vi "Test Modes.vi"(8 "error in (no error)":errorcluster, 11 "Instrument.Lockin in":refnum<class "Instrument.Lockin.lvclass">) -> (0 "error out":errorcluster, 3 "Instrument.Lockin out":refnum<class "Instrument.Lockin.lvclass">)   [LabVIEW 2016]
uses:
  src/Instrument.Lockin/Instrument.Lockin.lvclass
  src/Lockin.DAQ/Typedefs/AO_Channel-Numeric.ctl
  <vilib>/addons/_JKI Toolkits/Caraya/classes/Assert/Assert Equal Value_Variant.vi
  <vilib>/addons/_JKI Toolkits/Caraya/classes/Assert/Assert Not Error.vi
  <vilib>/addons/_JKI Toolkits/Caraya/classes/Assert/Assert Not Equal Value and Type_Variant.vi
  <vilib>/addons/_JKI Toolkits/Caraya/classes/Test/Test.lvclass
  <vilib>/addons/_JKI Toolkits/Caraya/classes/Assert/Assert.lvclass
  src/Lockin.DAQ/Lockin.DAQ.lvclass
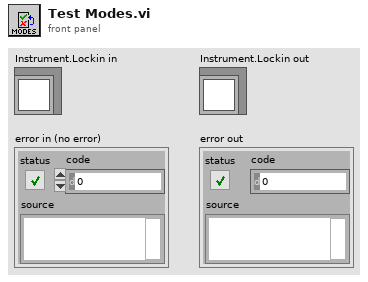
[diagram p1: front panel]
types:
  T1 = typedef "Lockin.DAQ.lvclass/AO_Channel-Numeric.ctl" = i32
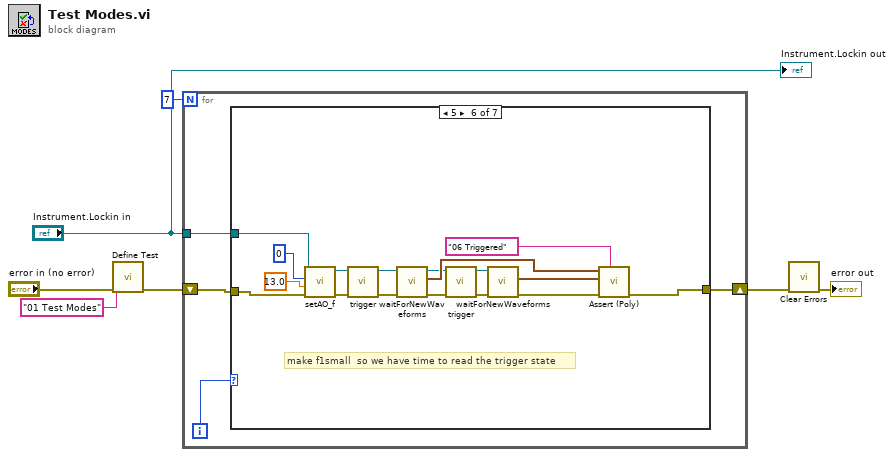
[diagram p0: block diagram]
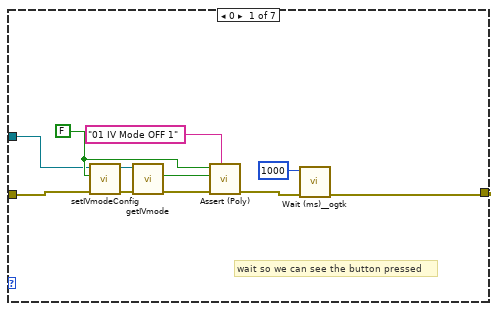
[diagram p2: hidden frame]
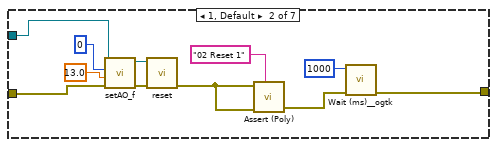
[diagram p3: hidden frame]
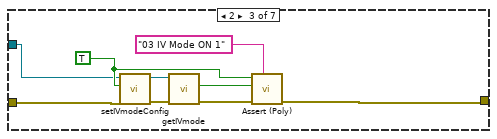
[diagram p4: hidden frame]
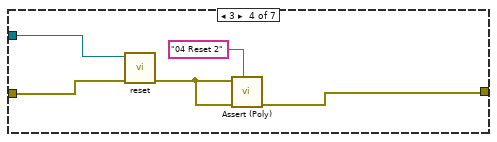
[diagram p5: hidden frame]
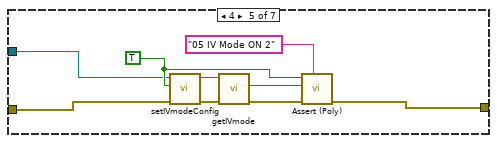
[diagram p6: hidden frame]
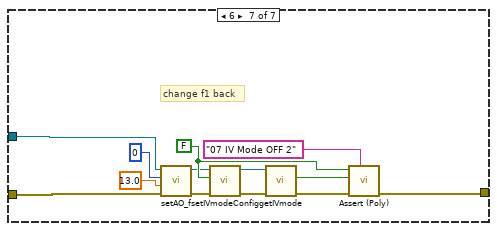
[diagram p7: hidden frame]
diagram:
  n1 = call <vilib>:"Define Test.vi"("error in (no error)"="error in (no error)", "Label (VI Title)"="01 Test Modes") -> ("error out"=w5:errorcluster)  [unwired: 9 in]
  n2 = for {
    N: 7 -> [_]
    tunnel: "Instrument.Lockin in" -> [w8]
    shift-right: [w9] -> w4
    shift-left: w5 -> [w10]
    i -> [w11]
    n3 = case shown="5" w11 {
      tunnel: w10 -> [w14 w28 w36 w46 w50 w59 w76]
      tunnel: [w12 w24 w34 w44 w48 w57 w74] -> w9
      tunnel: w8 -> [w13 w27 w35 w45 w49 w58 w75]
      frame 0 {
        w22 = FALSE ("IV mode")
        # "wait so we can see the button pressed"
        n4 = call "setIVmodeConfig.vi"("error in (no error)"=w14, "IV mode"=w22, "Instrument.Lockin in"=w13) -> ("error out"=w17:errorcluster, "Instrument.Lockin out"=w18:refnum<class "Instrument.Lockin.lvclass">)  [unwired: 7 in]
        n5 = call "getIVmode.vi"("error in (no error)"=w17, "Instrument.Lockin in"=w18) -> ("error out"=w19:errorcluster, "IV mode"=w21:bool)  [unwired: 7 in, 1 out]
        n6 = call-poly <vilib>:"Assert (Poly).vi"("Label"="01 IV Mode OFF 1", "error in (no error)"=w19, "Y"=w21, "X"=w22) -> ("error out"=w15:errorcluster)  [unwired: 7 in]
        n7 = call <userlib>:"Wait (ms)__ogtk.vi"("error in (no error)"=w15, "milliseconds to wait"=u32 1000) -> ("error out"=w12:errorcluster)  [unwired: 8 in, 1 out]
      }
      frame 1, Default {
        n8 = call "setAO_f.vi"("error in (no error)"=w28, "Frequency (Hz)"=13.0, "AO Channel"=T1 0, "Instrument.Lockin in"=w27) -> ("error out"=w32:errorcluster, "Instrument.Lockin out"=w33:refnum<class "Instrument.Lockin.lvclass">)  [unwired: 6 in]
        n9 = call "reset.vi"("error in (no error)"=w32, "Instrument.Lockin in"=w33) -> ("error out"=w23:errorcluster)  [unwired: 8 in, 1 out]
        n10 = call-poly <vilib>:"Assert (Poly).vi"("Label"="02 Reset 1", "error in (no error)"=w23, "Not Error?"=w23) -> ("error out"=w25:errorcluster)  [unwired: 8 in]
        n11 = call <userlib>:"Wait (ms)__ogtk.vi"("error in (no error)"=w25, "milliseconds to wait"=u32 1000) -> ("error out"=w24:errorcluster)  [unwired: 8 in, 1 out]
      }
      frame 2 {
        w42 = TRUE ("IV mode")
        n12 = call "setIVmodeConfig.vi"("error in (no error)"=w36, "IV mode"=w42, "Instrument.Lockin in"=w35) -> ("error out"=w38:errorcluster, "Instrument.Lockin out"=w37:refnum<class "Instrument.Lockin.lvclass">)  [unwired: 7 in]
        n13 = call "getIVmode.vi"("error in (no error)"=w38, "Instrument.Lockin in"=w37) -> ("error out"=w39:errorcluster, "IV mode"=w41:bool)  [unwired: 7 in, 1 out]
        n14 = call-poly <vilib>:"Assert (Poly).vi"("Label"="03 IV Mode ON 1", "error in (no error)"=w39, "Y"=w41, "X"=w42) -> ("error out"=w34:errorcluster)  [unwired: 7 in]
      }
      frame 3 {
        n15 = call "reset.vi"("error in (no error)"=w46, "Instrument.Lockin in"=w45) -> ("error out"=w43:errorcluster)  [unwired: 8 in, 1 out]
        n16 = call-poly <vilib>:"Assert (Poly).vi"("Label"="04 Reset 2", "error in (no error)"=w43, "Not Error?"=w43) -> ("error out"=w44:errorcluster)  [unwired: 8 in]
      }
      frame 4 {
        w51 = TRUE ("IV mode")
        n17 = call "setIVmodeConfig.vi"("error in (no error)"=w50, "IV mode"=w51, "Instrument.Lockin in"=w49) -> ("error out"=w55:errorcluster, "Instrument.Lockin out"=w56:refnum<class "Instrument.Lockin.lvclass">)  [unwired: 7 in]
        n18 = call "getIVmode.vi"("error in (no error)"=w55, "Instrument.Lockin in"=w56) -> ("error out"=w54:errorcluster, "IV mode"=w52:bool)  [unwired: 7 in, 1 out]
        n19 = call-poly <vilib>:"Assert (Poly).vi"("Label"="05 IV Mode ON 2", "error in (no error)"=w54, "Y"=w52, "X"=w51) -> ("error out"=w48:errorcluster)  [unwired: 7 in]
      }
      frame 5 {
        # "make f1small  so we have time to read the trigger state"
        n20 = call "setAO_f.vi"("error in (no error)"=w59, "Frequency (Hz)"=13.0, "AO Channel"=T1 0, "Instrument.Lockin in"=w58) -> ("error out"=w63:errorcluster, "Instrument.Lockin out"=w64:refnum<class "Instrument.Lockin.lvclass">)  [unwired: 6 in]
        n21 = call "trigger.vi"("error in (no error)"=w63, "Instrument.Lockin in"=w64) -> ("error out"=w65:errorcluster, "Instrument.Lockin out"=w66:refnum<class "Instrument.Lockin.lvclass">)  [unwired: 8 in]
        n22 = call "waitForNewWaveforms.vi"("error in (no error)"=w65, "Instrument.Lockin in"=w66) -> ("error out"=w67:errorcluster, "Newest AI Waveform"=w72:waveform(dbl)[], "Instrument.Lockin out"=w68:refnum<class "Instrument.Lockin.lvclass">)  [unwired: 7 in]
        n23 = call "trigger.vi"("error in (no error)"=w67, "Instrument.Lockin in"=w68) -> ("error out"=w69:errorcluster, "Instrument.Lockin out"=w70:refnum<class "Instrument.Lockin.lvclass">)  [unwired: 8 in]
        n24 = call "waitForNewWaveforms.vi"("error in (no error)"=w69, "Instrument.Lockin in"=w70) -> ("error out"=w73:errorcluster, "Newest AI Waveform"=w71:waveform(dbl)[])  [unwired: 7 in, 1 out]
        n25 = call-poly <vilib>:"Assert (Poly).vi"("Label"="06 Triggered", "error in (no error)"=w73, "Y"=w71, "X"=w72) -> ("error out"=w57:errorcluster)  [unwired: 7 in]
      }
      frame 6 {
        w85 = FALSE ("IV mode")
        # "change f1 back"
        n26 = call "setAO_f.vi"("error in (no error)"=w76, "Frequency (Hz)"=13.0, "AO Channel"=T1 0, "Instrument.Lockin in"=w75) -> ("error out"=w83:errorcluster, "Instrument.Lockin out"=w84:refnum<class "Instrument.Lockin.lvclass">)  [unwired: 6 in]
        n27 = call "setIVmodeConfig.vi"("error in (no error)"=w83, "IV mode"=w85, "Instrument.Lockin in"=w84) -> ("error out"=w78:errorcluster, "Instrument.Lockin out"=w77:refnum<class "Instrument.Lockin.lvclass">)  [unwired: 7 in]
        n28 = call "getIVmode.vi"("error in (no error)"=w78, "Instrument.Lockin in"=w77) -> ("error out"=w80:errorcluster, "IV mode"=w86:bool)  [unwired: 7 in, 1 out]
        n29 = call-poly <vilib>:"Assert (Poly).vi"("Label"="07 IV Mode OFF 2", "error in (no error)"=w80, "Y"=w86, "X"=w85) -> ("error out"=w74:errorcluster)  [unwired: 7 in]
      }
    }
  }
  n30 = call <vilib>:"Clear Errors.vi"("error in (no error)"=w4) -> ("error out"=→"error out":errorcluster)  [unwired: 5 in, 1 out]
  "Instrument.Lockin out" <- "Instrument.Lockin in"
